vi "init.vi"(8 "error in (no error)":errorcluster, 10 "Init Data":variant, 11 "Lakeshore 336 in":refnum<class "Lakeshore 336.lvclass">) -> (0 "error out":errorcluster, 2 "Channel List":refnum<class "HK Item.lvclass">[](array[class]), 3 "Lakeshore 336 out":refnum<class "Lakeshore 336.lvclass">)   [LabVIEW 2022 SP3, in "Lakeshore 336.lvclass"]
uses:
  Lakeshore 336.lvclass
  hk-channel-class/hk-channel-class/HK Item/HK Item.lvclass
  Lakeshore 336.lvclass/Lakeshore 336.ctl
  <instrlib>/Lake Shore 336/Lake Shore 336.lvlib
panel:
  out "Lake Shore 336 Address":refnum<visa-resource-name>="TCPIP0::192.168.121.12::7777::SOCKET"
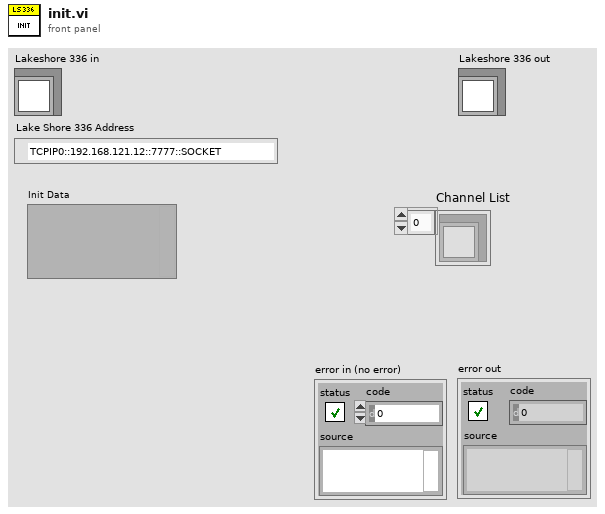
[diagram p1: front panel]
types:
  T1 = typedef "Lakeshore 336.lvclass/Lakeshore 336 Settings cluster.ctl" = cluster{"Lake Shore 336 Address":refnum<visa-resource-name>, "Output Ch":T2[], "Input Ch":T4[], "Prefix":string, "Setpoints":dbl[]}
  T2 = typedef "Lakeshore 336.lvclass/Lakeshore 336 Channel Settings cluster.ctl" = cluster{"Input (0:None)":u16, "Power Up Enable (F: Off)":bool, "Mode (0:Off)":u16, "Max Current (0:User Specified)":u16, "Heater Out Display (1:Current)":u16, "Max User Current (2.000)":dbl, "Heater Resistance (1:25 Ohms)":u16, "PID":T3, "Name":string}
  T3 = typedef "Lakeshore 336.lvclass/Lakeshore 336 PID cluster.ctl" = cluster{"P":dbl, "I":dbl, "D":dbl}
  T4 = typedef "Lakeshore 336.lvclass/Lakeshore 336 Input Ch config cluster.ctl" = cluster{"Name":string}
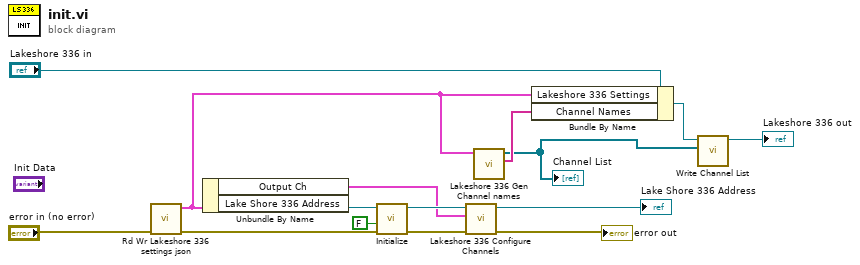
[diagram p0: block diagram]
diagram:
  n1 = call "Rd Wr Lakeshore 336 settings json.vi"("error in (no error)"="error in (no error)") -> ("error out"=w13:errorcluster, "Lakeshore 336 Settings"=w8:T1)  [unwired: 9 in]
  n2 = Unbundle By Name(w8) -> ("Output Ch"=w10:T2[], "Lake Shore 336 Address"=w14:refnum<visa-resource-name>)
  n3 = call <instrlib>:"Initialize.vi"("error in (no error)"=w13, "Reset (True)"=FALSE, "VISA resource name"=w14) -> ("error out"=w12:errorcluster, "VISA resource name out"=w11:refnum<visa-resource-name>)  [unwired: 7 in]
  n4 = call "Lakeshore 336 Configure Channels.vi"("error in"=w12, "Ch Setup"=w10, "VISA resource name"=w11) -> ("error out"=→"error out":errorcluster, "VISA resource name dup"=→"Lake Shore 336 Address":refnum<visa-resource-name>)  [unwired: 7 in]
  n5 = call "Lakeshore 336 Gen Channel names.vi"("Lakeshore 336 Settings"=w8) -> ("Channel Names"=w5:string[], "Channel List"=w3:refnum<class "HK Item.lvclass">[])  [unwired: 9 in]
  "Channel List" <- w3
  n6 = Bundle By Name(cluster="Lakeshore 336 in", "Lakeshore 336 Settings"=w8, "Channel Names"=w5) -> (w4:refnum<class "Lakeshore 336.lvclass">)
  n7 = call-dynamic "Write Channel List.vi"("Channel List"=w3, "Temp Control in"=w4) -> ("Temp Control out"=→"Lakeshore 336 out":refnum<class "Lakeshore 336.lvclass">)  [unwired: 8 in, 1 out]
